vi "UnloadModuleVisualization.vi"(8 "ErrorArray Out":errorcluster[](array[cluster]), 11 "Module Name in":string) -> (0 "ErrorArray":errorcluster[](array[cluster]), 1 "All Modules Stopped?":bool)   [LabVIEW 2018]
uses:
  VisualizationManagement/VisualizationManagerActions.ctl
  <userlib>/NIST/NISTErrorLib/NISTErrorLib.lvlib
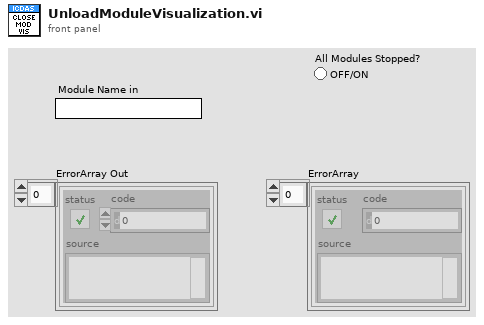
[diagram p1: front panel]
types:
  T1 = typedef "VisualizationManagerActions.ctl" = enum16{"Set", "LoadModVI", "PopInOutModVI", "Add", "Clear", "CloseVisMod", "LoadLatestModule", "Get"}
  T2 = typedef "cntlRefs.ctl" = cluster{"rngFGen":refnum<vi>, "rngDigitizer":refnum<vi>, "btnHide":refnum<vi>, "rngInst":refnum<vi>, "PluginTree":refnum<vi>, "TestListboxRef":refnum<vi>, "path.tstFile":refnum<vi>, "cmbxRunningModules":refnum<vi>, "TestDataSubPanel":refnum<vi>, "TestDataCaption":refnum<vi>, "btnPopInOut":refnum<vi>, "PluginMgrQ":refnum<queue>, "TestMgrQ":refnum<queue>, "TestMgrSubPanel":refnum<vi>, "PluginMgrSubPanel":refnum<vi>, "PwrReqHandle":u32, "btnStopOneTest":refnum<vi>, "pathUserfiles":refnum<vi>, "PluginTreeCaption":refnum<vi>, "MainVIRef":refnum<vi>, "btnStatus":refnum<vi>}
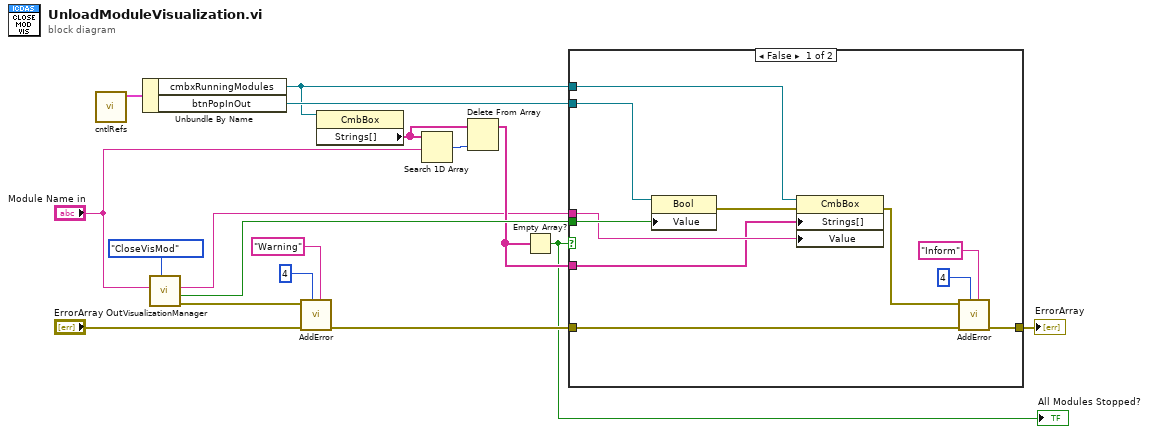
[diagram p0: block diagram]
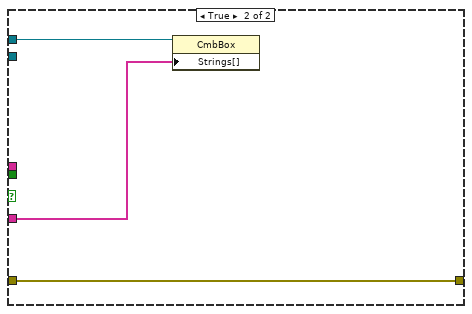
[diagram p2: hidden frame]
diagram:
  n1 = call "cntlRefs.vi"() -> ("cntlRefs"=w16:T2)  [unwired: 10 in, 1 out]
  n2 = Unbundle By Name(w16) -> ("cmbxRunningModules"=w7:refnum<vi>, "btnPopInOut"=w8:refnum<vi>)
  n3 = call "VisualizationManager.vi"("Action"=VisualizationManagerActions."CloseVisMod", "Module Name"="Module Name in") -> ("error out"=w11:errorcluster, "In SubPanel?"=w17:bool, "Module Name out"=w1:string)  [unwired: 6 in, 1 out]
  n4 = call <userlib>:"AddError.vi"("Severity"="Warning", "Priority"=u8 4, "ErrorArray In"="ErrorArray Out", "error in (no error)"=w11) -> ("ErrorArray Out"=w14:errorcluster[])  [unwired: 6 in, 1 out]
  n5 = property class="CmbBox"(reference=w7) -> ("Strings[]"=w5:string[])  [unwired: 1 in, 2 out]
  n6 = Search 1D Array(1D array=w5, element="Module Name in") -> (index of element=w6:i32)  [unwired: 1 in]
  n7 = Delete From Array(array=w5, index=w6) -> (array with subset deleted=w4:string[])  [unwired: 1 in, 1 out]
  n8 = Empty Array?(array=w4) -> (empty?=w3:bool)
  "All Modules Stopped?" <- w3
  n9 = case shown="False" w3 {
    tunnel: w14 -> [w18 w31]
    tunnel: [w19 w31] -> w15
    tunnel: w7 -> [w28 w30]
    tunnel: w8 -> [w27 _]
    tunnel: w17 -> [w26 _]
    tunnel: w1 -> [w25 _]
    tunnel: w4 -> [w24 w29]
    frame False {
      n10 = property class="Bool"(reference=w27, "Value"=w26) -> (error out=w23:errorcluster)  [unwired: 1 in, 1 out]
      n11 = property class="CmbBox"(reference=w28, error in=w23, "Strings[]"=w24, "Value"=w25) -> (error out=w20:errorcluster)  [unwired: 1 out]
      n12 = call <userlib>:"AddError.vi"("Severity"="Inform", "Priority"=u8 4, "ErrorArray In"=w18, "error in (no error)"=w20) -> ("ErrorArray Out"=w19:errorcluster[])  [unwired: 6 in, 1 out]
    }
    frame True {
      n13 = property class="CmbBox"(reference=w30, "Strings[]"=w29) -> ()  [unwired: 1 in, 2 out]
    }
  }
  "ErrorArray" <- w15
